vi "free enumerate.vi"(8 "error in (no error)":errorcluster, 11 "para0":cluster{}) -> (0 "error out":errorcluster, 3 "para0 out":cluster{})   [LabVIEW 2022 SP3, in "usb_relay_device.lvlib"]
doc: "void EXPORT_API usb_relay_device_free_enumerate(struct usb_relay_device_info*);"
uses:
  usb_relay_device.lvlib
  AppBuilderFiles/RunTimeExe/data/usb_relay_device.dll
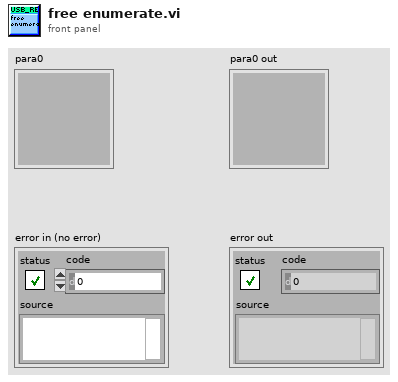
[diagram p1: front panel]
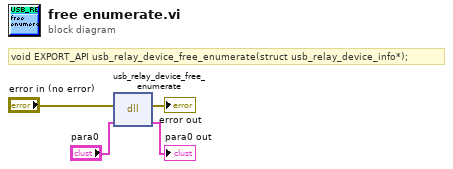
[diagram p0: block diagram]
diagram:
  # "void EXPORT_API usb_relay_device_free_enumerate(struct usb_relay_device_info*);"
  n1 = dll-call lib="D:/LabVIEWSuite_64_OS/AppBuilderFiles/RunTimeExe/data/usb_relay_device.*" fn="usb_relay_device_free_enumerate"(error in="error in (no error)", "para0"="para0") -> (error out=→"error out":errorcluster, "para0"=→"para0 out":cluster{})  [unwired: 3 in, 1 out]
